vi "Resolve-message-type.vi"(8 "error in (no error)":errorcluster, 11 "Message":refnum<class "Message.lvclass">) -> (0 "error out":errorcluster, 2 "Message type":T1, 3 "Message dup":refnum<class "Message.lvclass">)   [LabVIEW 2013, in "PowderDeposition.lvlib" / "PD-Client.lvclass"]
uses:
  PD-Client.lvclass
  SA-SLMAPI/Sources/Message.lvclass
  Supported-messages.ctl
  SA-SLMAPI/Sources/Message.lvclass/Message.ctl
  Custom-errors.ctl
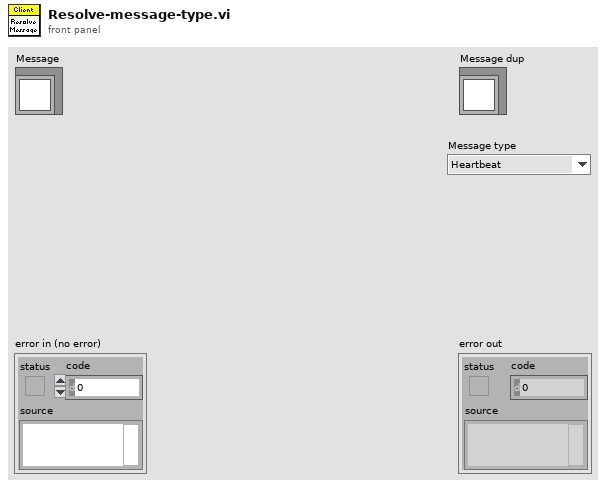
[diagram p1: front panel]
types:
  T1 = typedef "PowderDeposition.lvlib/PD-Client.lvclass/Supported-messages.ctl" = enum16{"Heartbeat", "Error", "Client stopped", "Action", "Query status", "Send status", "Get clients"}
  T2 = typedef "PowderDeposition.lvlib/PD-Client.lvclass/Custom-errors.ctl" = enum16{"No error", "Command not recognized", "Invalid input", "Timeout", "Not implemented", "Unsupported message", "Unsupported client", "Unsupported action"}
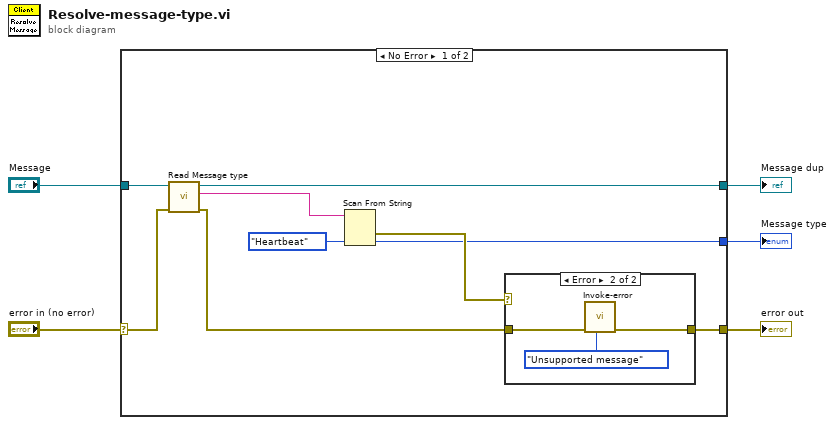
[diagram p0: block diagram]
diagram:
  n1 = case shown="No Error" "error in (no error)" {
    selector: "error in (no error)" -> [w10 w20]
    tunnel: [w7 w20] -> w4
    tunnel: "Message" -> [w14 w19]
    tunnel: [w13 w19] -> w2
    tunnel: [w6 _] -> w1
    frame No Error {
      n2 = call "Read Message type.vi"("error in (no error)"=w10, "Message in"=w14) -> ("error out"=w8:errorcluster, "String"=w11:string, "Message out"=w13:refnum<class "Message.lvclass">)  [unwired: 7 in]
      n3 = Scan From String(input string=w11, default 1=Supported-messages."Heartbeat" ("Type")) -> (error out=w9:errorcluster, output 1=w6:T1)  [unwired: 3 in, 2 out]
      n4 = case shown="Error" w9 {
        tunnel: w8 -> [w15 w17]
        tunnel: [w15 w16] -> w7
        frame No Error {
        }
        frame Error {
          n5 = call "Invoke-error.vi"("Error"=Custom-errors."Unsupported message", "error in (no error)"=w17) -> ("error out"=w16:errorcluster)  [unwired: 9 in]
        }
      }
    }
    frame Error {
    }
  }
  "error out" <- w4
  "Message dup" <- w2
  "Message type" <- w1
